vi "Create Python Graph (Example).vi"() -> ()   [LabVIEW 2013]
panel:
  out "Error OUT":errorcluster
  out "Command Line Error":string
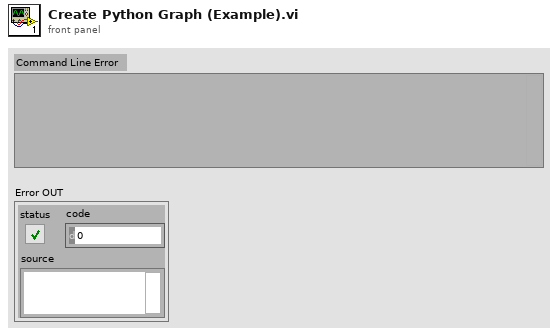
[diagram p1: front panel]
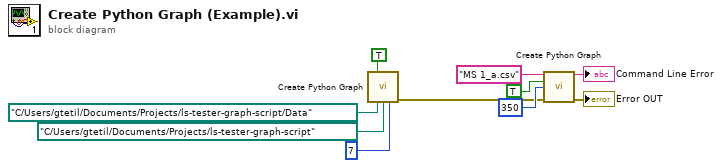
[diagram p0: block diagram]
diagram:
  n1 = call "Create Python Graph.vi"("Init (F)"=TRUE, "Data Base Path"=path "C:/Users/gtetil/Documents/Projects/ls-tester-graph-script/Data", "Python Script Directory"=path "C:/Users/gtetil/Documents/Projects/ls-tester-graph-script", "Data Start Index"=u32 7) -> ("Error OUT"=w6:errorcluster)  [unwired: 10 in, 1 out]
  n2 = call "Create Python Graph.vi"("File Name"="MS 1_a.csv", "Wet Test"=TRUE, "Y-Axis Max"=350, "Error IN"=w6) -> ("Command Line Error"=→"Command Line Error":string, "Error OUT"=→"Error OUT":errorcluster)  [unwired: 10 in]
